vi "init_quiver.vi"(9 "XY Spacing":dbl format="%#_13g", 10 "Cols":i32, 11 "Rows":i32) -> (2 "Quiver Data Prealloc":dbl[][](array[numeric]), 3 "Quiver Grid":dbl[][](array[numeric]))   [LabVIEW 2016]
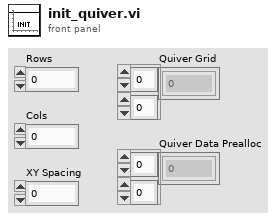
[diagram p1: front panel]
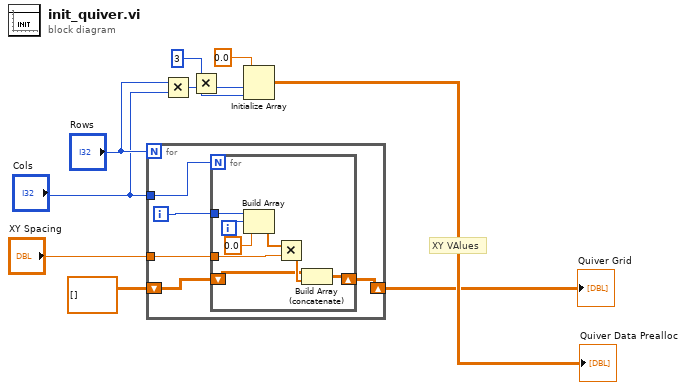
[diagram p0: block diagram]
diagram:
  w9 = 3
  # "XY VAlues"
  n1 = for {
    N: "Rows" -> [_]
    tunnel: "Cols" -> [w15]
    tunnel: "XY Spacing" -> [w14]
    shift-right: [w12] -> w3
    shift-left: dbl[][] [] ("x*y") -> [w11]
    i -> [w13]
    n2 = for {
      N: w15 -> [_]
      tunnel: w14 -> [w21]
      tunnel: w13 -> [w22]
      shift-right: [w18] -> w12
      shift-left: w11 -> [w17]
      i -> [w23]
      n3 = Build Array(w22, w23, 0.0) -> (w20:dbl[])
      n4 = Multiply(x=w20, y=w21) -> (x*y=w19:dbl[])
      n5 = Build Array (concatenate)(w17, w19) -> (w18:dbl[][])
    }
  }
  "Quiver Grid" <- w3
  n6 = Multiply(x="Rows", y="Cols") -> (x*y=w6:i32)
  n7 = Multiply(x=w9, y=w6) -> (x*y=w7:i32)
  n8 = Initialize Array(0.0, w7, w9) -> (→"Quiver Data Prealloc":dbl[][])
